vi "Untitled 3.vi"() -> ()   [LabVIEW 2017]
uses:
  <vilib>/rvi/DataTransferAndStorage/Container/XNode/niFpgaContainer.xnode
  <vilib>/rvi/FIFO/Fifo_Resource/niFpgaFifoEmulationRefIn.vi
panel:
  in  "FIFO In":refnum<k21>="FIFO"
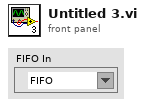
[diagram p1: front panel]
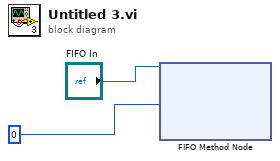
[diagram p0: block diagram]
diagram:
  n1 = xnode ("FIFO Method Node")("Element"=i16 0, "FIFO In"="FIFO In") -> ()  [unwired: 1 in, 2 out]
